vi "APPA109N - Read.vi"(11 "VISA resource name":refnum<visa-resource-name>) -> (0 "error out":errorcluster, 1 "Units":T1(ring), 2 "Number":dbl, 3 "VISA resource name out":refnum<visa-resource-name>, 4 "Number (sub-panel)":dbl, 5 "Regime":string, 6 "Checksum":bool)   [LabVIEW 2016]
panel:
  in  "error in (no error)":errorcluster
  # "Press button while turning meter on from OFF position.\nRANGE : Turn off beeper.\nBLUE : Disable Auto Power OFF."
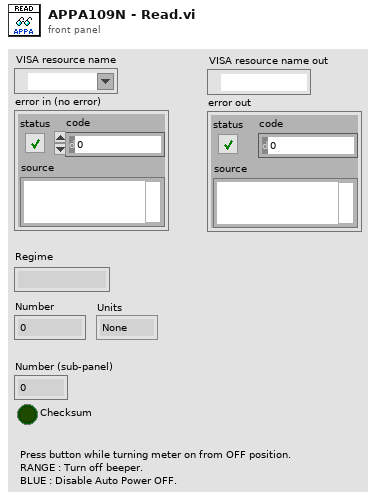
[diagram p1: front panel]
types:
  T1 = enum16{"None", "V", "mV", "A", "mA", "dB", "dBm", "nF", "uF", "mF", "Ohm", "kOhm", "MOhm", "GOhm", "%", "Hz", "kHz", "MHz", "C", "F", "s", "ms", "ns", "V (manual)", "mV (manual)", "A (manual)", "mA (manual)", "Ohm (manual)", "kOhm (maual)", "MOhm (manual)", ""}
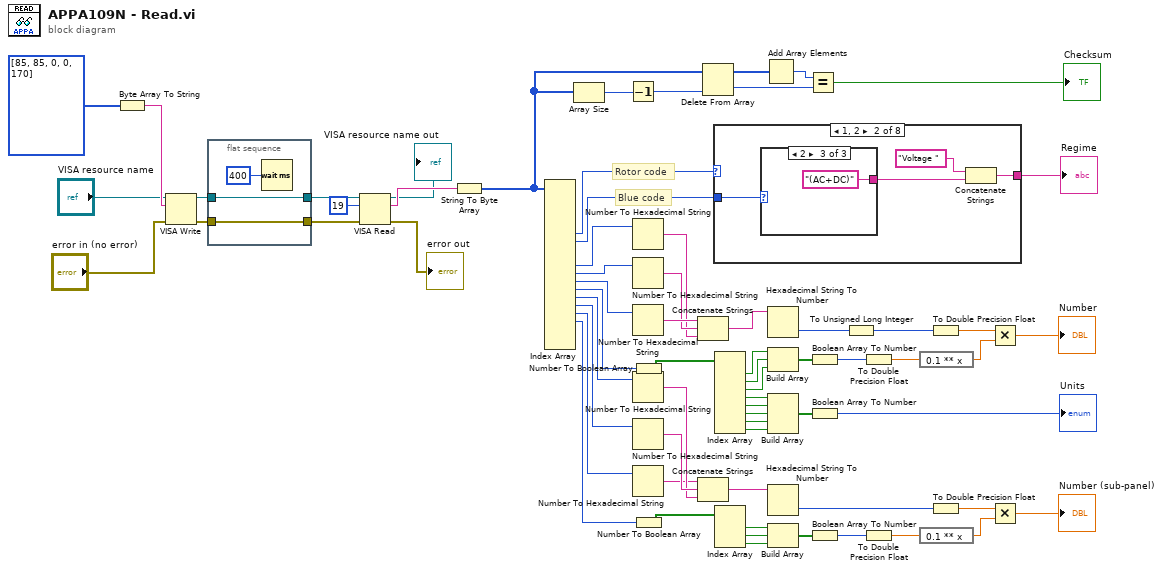
[diagram p0: block diagram]
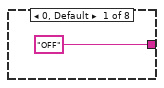
[diagram p2: hidden frame]
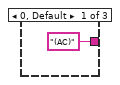
[diagram p3: hidden frame]
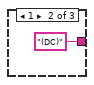
[diagram p4: hidden frame]
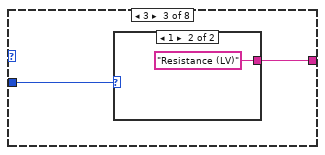
[diagram p5: hidden frame]
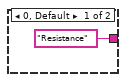
[diagram p6: hidden frame]
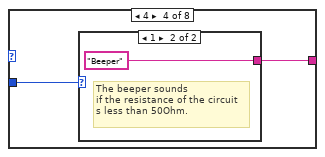
[diagram p7: hidden frame]
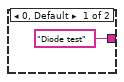
[diagram p8: hidden frame]
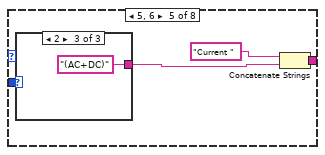
[diagram p9: hidden frame]
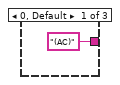
[diagram p10: hidden frame]
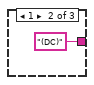
[diagram p11: hidden frame]
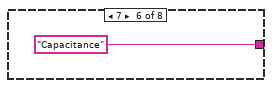
[diagram p12: hidden frame]
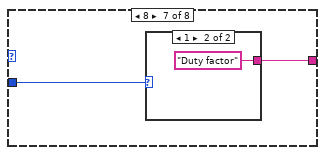
[diagram p13: hidden frame]
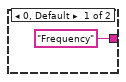
[diagram p14: hidden frame]
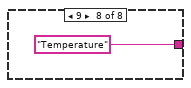
[diagram p15: hidden frame]
diagram:
  # "Blue code"
  # "Rotor code"
  n1 = Byte Array To String(unsigned byte array=i32[] [85, 85, 0, 0, 170]) -> (string=w62:string)
  n2 = VISA Write(VISA resource name="VISA resource name", write buffer=w62, error in (no error)="error in (no error)") -> (VISA resource name out=w68:refnum<visa-resource-name>, error out=w67:errorcluster)  [unwired: 1 out]
  n3 = flat-sequence {
    tunnel: w68 -> [w70]
    tunnel: w67 -> [w69]
    tunnel: [w70] -> w66
    tunnel: [w69] -> w65
    frame #0 {
      n4 = Wait (ms)(milliseconds to wait=u32 400) -> ()  [unwired: 1 out]
    }
  }
  n5 = VISA Read(VISA resource name=w66, byte count=u32 19, error in (no error)=w65) -> (VISA resource name out=→"VISA resource name out":refnum<visa-resource-name>, read buffer=w61:string, error out=→"error out":errorcluster)  [unwired: 1 out]
  n6 = String To Byte Array(string=w61) -> (unsigned byte array=w34:u8[])
  n7 = Index Array(array=w34) -> (element #5=w60:u8, element #6=w59:u8, element #9=w56:u8, element #10=w57:u8, element #11=w58:u8, element #12=w51:u8, element #13=w23:u8, element #14=w22:u8, element #15=w21:u8, element #16=w12:u8)  [unwired: 19 in, 9 out]
  n8 = Array Size(array=w34) -> (size(s)=w35:i32)
  n9 = Decrement(x=w35) -> (x-1=w33:i32)
  n10 = Number To Hexadecimal String(2:w56) -> (0:w53:string)  [unwired: 1 in]
  n11 = Number To Hexadecimal String(2:w57) -> (0:w54:string)  [unwired: 1 in]
  n12 = Number To Hexadecimal String(2:w58) -> (0:w55:string)  [unwired: 1 in]
  n13 = Number To Hexadecimal String(2:w23) -> (0:w28:string)  [unwired: 1 in]
  n14 = Number To Hexadecimal String(2:w22) -> (0:w29:string)  [unwired: 1 in]
  n15 = Number To Hexadecimal String(2:w21) -> (0:w24:string)  [unwired: 1 in]
  n16 = Number To Boolean Array(number=w51) -> (Boolean array=w50:bool[])
  n17 = Number To Boolean Array(number=w12) -> (Boolean array=w20:bool[])
  n18 = Concatenate Strings(w55, w54, w53) -> (w52:string)
  n19 = Concatenate Strings(w24, w29, w28) -> (w27:string)
  n20 = Delete From Array(array=w34, index=w33) -> (deleted portion=w30:u8, array with subset deleted=w32:u8[])  [unwired: 1 in]
  n21 = case shown="1, 2" w60 {
    tunnel: ["OFF" w74 w81 w84 w88 "Capacitance" w96 "Temperature"] -> w9
    tunnel: w59 -> [_ w76 w80 w85 w90 _ w97 _]
    frame 0, Default {
    }
    frame 1, 2 {
      n22 = case shown="2" w76 {
        tunnel: ["(AC)" "(DC)" "(AC+DC)"] -> w73
        frame 0, Default {
        }
        frame 1 {
        }
        frame 2 {
        }
      }
      n23 = Concatenate Strings("Voltage ", w73) -> (w74:string)
    }
    frame 3 {
      n24 = case shown="1" w80 {
        tunnel: ["Resistance" "Resistance (LV)"] -> w81
        frame 0, Default {
        }
        frame 1 {
        }
      }
    }
    frame 4 {
      n25 = case shown="1" w85 {
        tunnel: ["Diode test" "Beeper"] -> w84
        frame 0, Default {
        }
        frame 1 {
          # "The beeper sounds\nif the resistance of the circuit\ns less than 50Ohm."
        }
      }
    }
    frame 5, 6 {
      n26 = case shown="2" w90 {
        tunnel: ["(AC)" "(DC)" "(AC+DC)"] -> w91
        frame 0, Default {
        }
        frame 1 {
        }
        frame 2 {
        }
      }
      n27 = Concatenate Strings("Current ", w91) -> (w88:string)
    }
    frame 7 {
    }
    frame 8 {
      n28 = case shown="1" w97 {
        tunnel: ["Frequency" "Duty factor"] -> w96
        frame 0, Default {
        }
        frame 1 {
        }
      }
    }
    frame 9 {
    }
  }
  "Regime" <- w9
  n29 = Index Array(array=w50) -> (element #1=w49:bool, element #2=w48:bool, element #3=w47:bool, element #4=w41:bool, element #5=w40:bool, element #6=w39:bool, element #7=w38:bool, element #8=w37:bool)  [unwired: 8 in]
  n30 = Index Array(array=w20) -> (element #1=w19:bool, element #2=w18:bool, element #3=w17:bool)  [unwired: 3 in]
  n31 = Add Array Elements(numeric array=w32) -> (sum=w31:u8)
  n32 = Hexadecimal String To Number(string=w52) -> (number=w1:u32)  [unwired: 2 in, 1 out]
  n33 = Build Array(w49, w48, w47) -> (w46:bool[])
  n34 = Build Array(w41, w40, w39, w38, w37) -> (w36:bool[])
  n35 = Hexadecimal String To Number(string=w27) -> (number=w26:u32)  [unwired: 2 in, 1 out]
  n36 = Build Array(w19, w18, w17) -> (w16:bool[])
  n37 = Equal?(x=w31, y=w30) -> (x = y?=→"Checksum":bool)
  n38 = Boolean Array To Number(Boolean array=w46) -> (number=w45:u32)
  n39 = Boolean Array To Number(Boolean array=w36) -> (number=→"Units":u32)
  n40 = Boolean Array To Number(Boolean array=w16) -> (number=w15:u32)
  n41 = To Unsigned Long Integer(number=w1) -> (unsigned 32bit integer=w2:u32)
  n42 = To Double Precision Float(number=w45) -> (double precision float=w43:dbl)
  n43 = To Double Precision Float(number=w15) -> (double precision float=w14:dbl)
  n44 = expression code="0.1 ** x"(w43) -> (w42:dbl)
  n45 = expression code="0.1 ** x"(w14) -> (w13:dbl)
  n46 = To Double Precision Float(number=w2) -> (double precision float=w44:dbl)
  n47 = To Double Precision Float(number=w26) -> (double precision float=w25:dbl)
  n48 = Multiply(x=w44, y=w42) -> (x*y=→"Number":dbl)
  n49 = Multiply(x=w25, y=w13) -> (x*y=→"Number (sub-panel)":dbl)
